vi "AlazarAbortCapture.vi"(0 "Handle":u32, 1 "error in (no error)":errorcluster) -> (2 "Handle":u32, 3 "Return Code":u32, 4 "error out":errorcluster)   [LabVIEW 2021]
doc: "Abort an acquisition to on-board memory."
uses:
  ATSApi.dll
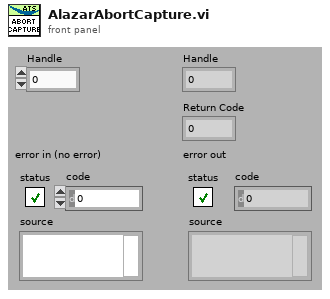
[diagram p1: front panel]
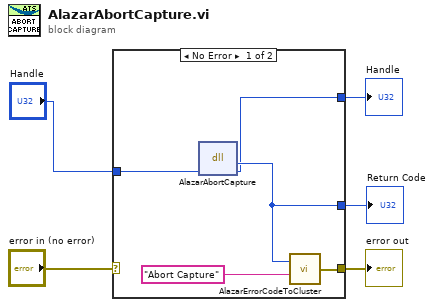
[diagram p0: block diagram]
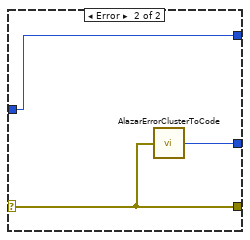
[diagram p2: hidden frame]
diagram:
  n1 = case shown="No Error" "error in (no error)" {
    selector: "error in (no error)" -> [_ w13]
    tunnel: [w7 w13] -> w4
    tunnel: [w9 w12] -> w3
    tunnel: "Handle" -> [w10 w11]
    tunnel: [w6 w11] -> w1
    frame No Error {
      n2 = dll-call lib="ATSApi.dll" fn="AlazarAbortCapture"("handle"=w10) -> (w9:u32, "handle"=w6:u32)  [unwired: 3 in, 2 out]
      n3 = call "AlazarErrorCodeToCluster.vi"("Message"="Abort Capture", "Error Code"=w9) -> ("error out"=w7:errorcluster)
    }
    frame Error {
      n4 = call "AlazarErrorClusterToCode.vi"("error in (no error)"=w13) -> ("Error Code"=w12:u32)
    }
  }
  "Handle" <- w1
  "error out" <- w4
  "Return Code" <- w3
